vi "Create Trigger Model Place Holder Block.vi"(0 "VISA resource name":refnum<visa-resource-name>, 5 "Block Number (1)":i32=1 min=1 format="%#.6g", 11 "error in (no error)":errorcluster) -> (4 "VISA resource name out":refnum<visa-resource-name>, 15 "error Out (no error)":errorcluster)   [LabVIEW 2018, in "Keithley DMM7512.lvlib"]
doc: "This VI creates a placeholder that performs no action in the trigger model."
uses:
  <instrlib>/Keithley DMM7512/Keithley DMM7512.lvlib
panel:
  # "NOTE: in this vi one parameter called logic i have not implemented once\nthe new manual comes check the example in that and implement it -Shashi"
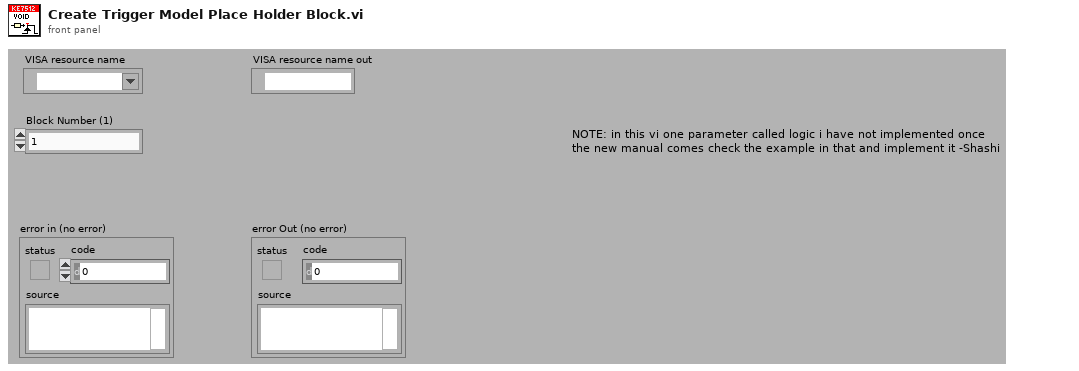
[diagram p1: front panel]
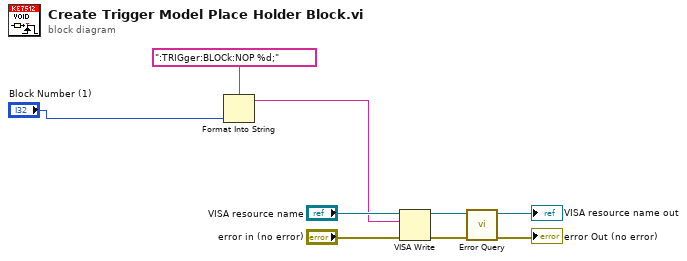
[diagram p0: block diagram]
diagram:
  n1 = Format Into String(format string=":TRIGger:BLOCk:NOP %d;", "Block Number (1)") -> (resulting string=w6:string)  [unwired: 2 in, 1 out]
  n2 = VISA Write(VISA resource name="VISA resource name", write buffer=w6, error in (no error)="error in (no error)") -> (VISA resource name out=w5:refnum<visa-resource-name>, error out=w3:errorcluster)  [unwired: 1 out]
  n3 = call <instrlib>:"Error Query.vi"("error in (no error)"=w3, "VISA resource name"=w5) -> ("error out"=→"error Out (no error)":errorcluster, "VISA resource name out"=→"VISA resource name out":refnum<visa-resource-name>)  [unwired: 6 in, 2 out]
